vi "Register Form FKs.vi"(8 "error in (no error)":errorcluster, 9 "FK/PK Info":T1, 10 "Form ID":T2, 11 "Form Server in":refnum<class "Form Server.lvclass">) -> (0 "error out":errorcluster, 3 "Form Server out":refnum<class "Form Server.lvclass">)   [LabVIEW 2020, in "Form Server.lvlib" / "Form Server.lvclass"]
uses:
  Form Server.lvclass
  Autoclose manager/Form ID.ctl
  Update Fields Logic/Field FK PK Info.ctl
  Form Server.lvclass/Form Server.ctl
  Form Server Configuration/Form Server Configuration.lvclass/Form Server Configuration.ctl
  Update Fields Logic/Update Fields Logic.lvclass
  Form Server Configuration/Form Server Configuration.lvclass
  Form Server Interfaces.lvlib
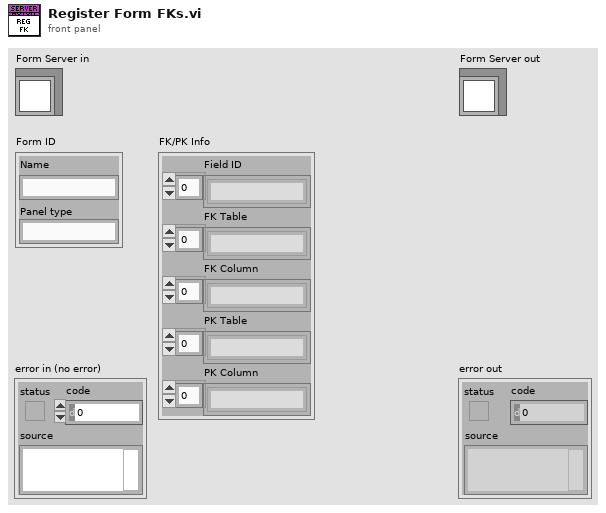
[diagram p1: front panel]
types:
  T1 = typedef "Form Server Interfaces.lvlib/Field FK PK Info.ctl" = cluster{"Field ID":string[], "FK Table":string[], "FK Column":string[], "PK Table":string[], "PK Column":string[]}
  T2 = typedef "Form Server Interfaces.lvlib/Form ID.ctl" = cluster{"Name":string, "Panel type":string}
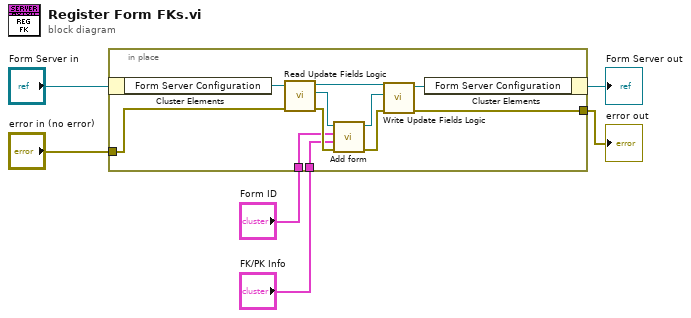
[diagram p0: block diagram]
diagram:
  n1 = in-place {
    in-place-border: [w11] -> w4
    in-place-border: "error in (no error)" -> [w10]
    in-place-border: "Form ID" -> [w8]
    in-place-border: "FK/PK Info" -> [w7]
    n2 = in-place-cluster #1("Form Server in") -> ("Form Server Configuration"=w17:refnum<class "Form Server Configuration.lvclass">)
    n3 = call "Read Update Fields Logic.vi"("error in (no error)"=w10, "Form Server Configuration in"=w17) -> ("error out"=w9:errorcluster, "Form Server Interfaces.lvlib:Update Fields Logic.lvclass"=w14:refnum<class "Update Fields Logic.lvclass">, "Form Server Configuration out"=w16:refnum<class "Form Server Configuration.lvclass">)  [unwired: 7 in]
    n4 = call-dynamic "Add form.vi"("error in (no error)"=w9, "FK/PK Info"=w7, "Form ID"=w8, "Update Fields Logic in"=w14) -> ("error out"=w12:errorcluster, "Update Fields Logic out"=w13:refnum<class "Update Fields Logic.lvclass">)  [unwired: 5 in, 1 out]
    n5 = call "Write Update Fields Logic.vi"("error in (no error)"=w12, "Form Server Interfaces.lvlib:Update Fields Logic.lvclass"=w13, "Form Server Configuration in"=w16) -> ("error out"=w11:errorcluster, "Form Server Configuration out"=w15:refnum<class "Form Server Configuration.lvclass">)  [unwired: 7 in]
    n6 = in-place-cluster #1("Form Server Configuration"=w15) -> (→"Form Server out":refnum<class "Form Server.lvclass">)
  }
  "error out" <- w4
